vi "BeginFinishold.vi"(11 "Enum":enum16{"Start", "Run", "End"}(ring)) -> ()   [LabVIEW 2012]
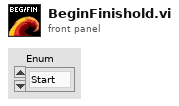
[diagram p1: front panel]
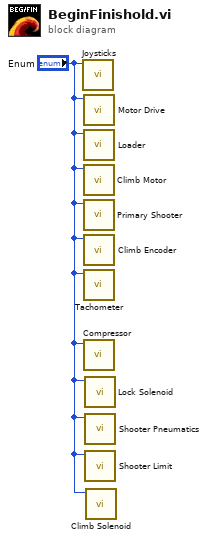
[diagram p0: block diagram]
diagram:
  n1 = call "Joysticks.vi"("Enum"="Enum") -> ()  [unwired: 9 in, 2 out]
  n2 = call "Motor Drive.vi"("Enum"="Enum") -> ()  [unwired: 11 in]
  n3 = call "Loader.vi"("Enum"="Enum") -> ()  [unwired: 10 in]
  n4 = call "Climb Motor.vi"("Enum"="Enum") -> ()  [unwired: 11 in]
  n5 = call "Primary Shooter.vi"("Enum"="Enum") -> ()  [unwired: 11 in]
  n6 = call "Climb Encoder.vi"("Enum"="Enum") -> ()  [unwired: 10 in, 1 out]
  n7 = call "Tachometer.vi"("Enum"="Enum") -> ()  [unwired: 10 in, 1 out]
  n8 = call "Compressor.vi"("Enum"="Enum") -> ()  [unwired: 11 in]
  n9 = call "Lock Solenoid.vi"("Enum"="Enum") -> ()  [unwired: 11 in]
  n10 = call "Shooter Pneumatics.vi"("Enum"="Enum") -> ()  [unwired: 10 in, 1 out]
  n11 = call "Shooter Limit.vi"("Enum"="Enum") -> ()  [unwired: 10 in, 1 out]
  n12 = call "Climb Solenoid.vi"("Enum"="Enum") -> ()  [unwired: 11 in]
